vi "Create file reference.vi"(8 "error in (no error)":errorcluster) -> (0 "error out":errorcluster, 3 "File reference":refnum<file>)   [LabVIEW 2020]
uses:
  <vilib>/Utility/sysdir.llb/System Directory Type.ctl
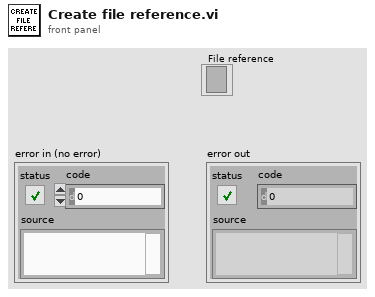
[diagram p1: front panel]
types:
  T1 = typedef "System Directory Type.ctl" = i32
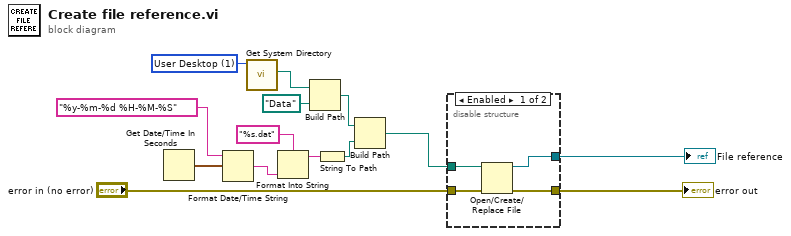
[diagram p0: block diagram]
diagram:
  w8 = T1 1 items=["User Home"=0, "User Desktop"=1, "User Documents"=2, "User Application Data"=3, "User Preferences"=4, "User Temporary"=5, "Public Documents"=6, "Public Application Data"=7, "Public Preferences"=8, "Public Cache"=13, "System Core Libraries"=9, "System Installed Libraries"=10, "Application Files"=11, "Boot Volume Root"=12] ("system directory type")
  n1 = Get Date/Time In Seconds() -> (seconds since 1Jan1904=w1:timestamp)
  n2 = Format Date/Time String(time format string (%c)="%y-%m-%d %H-%M-%S", seconds (now)=w1) -> (date/time string=w5:string)  [unwired: 1 in]
  n3 = call <vilib>:"Get System Directory.vi"("system directory type"=w8) -> ("system directory"=w10:path)  [unwired: 10 in]
  n4 = Format Into String(format string="%s.dat", w5) -> (resulting string=w3:string)  [unwired: 2 in, 1 out]
  n5 = Build Path(base path=w10, name or relative path=path "Data") -> (appended path=w13:path)
  n6 = String To Path(string=w3) -> (path=w2:path)
  n7 = Build Path(base path=w13, name or relative path=w2) -> (appended path=w14:path)
  n8 = disable-structure shown="Enabled" {
    disable-tunnel: w14 -> [w18 _]
    disable-tunnel: "error in (no error)" -> [w17 w19]
    disable-tunnel: [w16 _] -> w9
    disable-tunnel: [w15 w19] -> w7
    frame Enabled {
      n9 = Open/Create/Replace File(file path (use dialog)=w18, error in=w17) -> (refnum out=w16:refnum<file>, error out=w15:errorcluster)  [unwired: 4 in, 1 out]
    }
    frame Disabled {
    }
  }
  "File reference" <- w9
  "error out" <- w7
